vi "Number of Events Global.vi"() -> ()   [LabVIEW 2016]
panel:
  out "Number of Events":i32
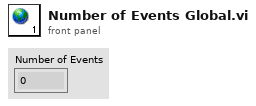
[diagram p1: front panel]
diagram:
